vi "Temperature On Error.vi"() -> ()   [LabVIEW 2012, in "Phidget Temperature Sensor.lvlib"]
uses:
  <instrlib>/Phidgets/Phidget Temperature Sensor/Phidget Temperature Sensor.lvlib
  <instrlib>/Phidgets/Phidget Temperature Sensor/Public/TemperatureSensorStart.vi
  <instrlib>/Phidgets/Phidget Temperature Sensor/Public/TemperatureSensorClose.vi
  <instrlib>/Phidgets/Phidget Common/Phidget Common.lvlib
panel:
  out "Serial Number Return":i32
  in  "Device Info":T1={"Serial Number"=-1, "Channel"=0, "Port"=0}
  out "error out":errorcluster
  in  "stop":bool
  out "ErrorString":string
  out "ErrorCode":i32
  # "This will receive the error generated if a reading is out of range"
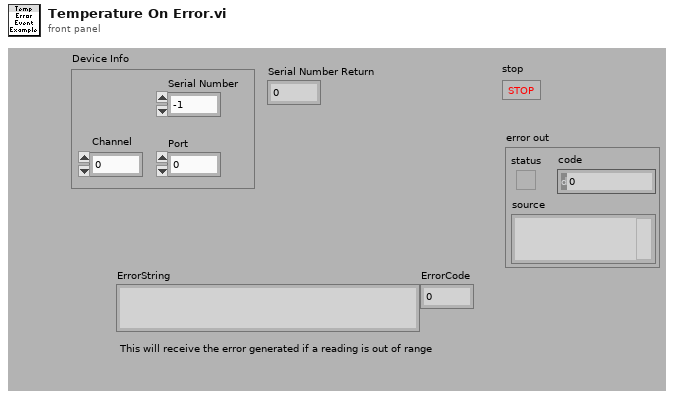
[diagram p1: front panel]
types:
  T1 = cluster{"Serial Number":i32, "Channel":i32, "Port":i32}
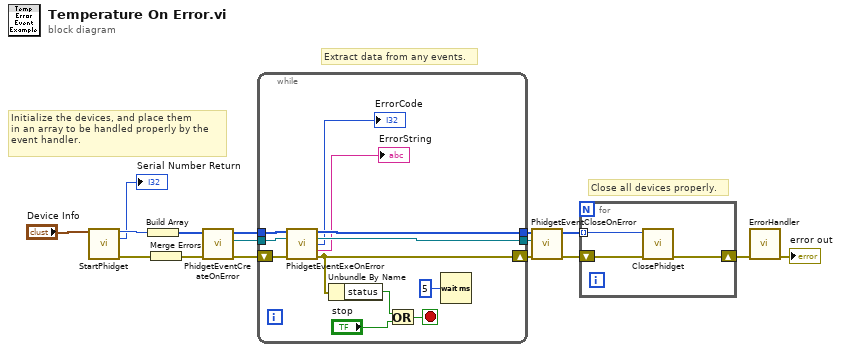
[diagram p0: block diagram]
diagram:
  # "Close all devices properly."
  # "Extract data from any events."
  # "Initialize the devices, and place them\nin an array to be handled properly by the\nevent handler."
  n1 = call-poly <instrlib>:"StartPhidget.vi"("Device Info"="Device Info") -> ("Phidget ID"=w5:u64, "Serial Number Return"=→"Serial Number Return":i32, "error out"=w1:errorcluster)  [unwired: 11 in, 1 out]
  n2 = Build Array(w5) -> (w16:u64[])
  n3 = Merge Errors(w1) -> (w7:errorcluster)
  n4 = call <instrlib>:"PhidgetEventCreateOnError.vi"("error in (no error)"=w7, "Devices In"=w16) -> ("error out"=w9:errorcluster, "Event Registration Refnum"=w14:refnum<event-registration>, "Devices Out"=w15:u64[])  [unwired: 7 in]
  n5 = while {
    tunnel: w15 -> [w28]
    tunnel: w14 -> [w24]
    tunnel: [w27] -> w11
    shift-right: [w17] -> w10
    shift-left: w9 -> [w26]
    tunnel: [w20] -> w3
    stop <- w23 stop-if-true
    n6 = call <instrlib>:"PhidgetEventExeOnError.vi"("Devices In"=w28, "Event Registration Refnum In"=w24, "error in (no error)"=w26) -> ("Devices Out"=w20:u64[], "Event Registration Refnum Out"=w27:refnum<event-registration>, "ErrorCode"=→"ErrorCode":i32, "ErrorString"=→"ErrorString":string, "error out"=w17:errorcluster)  [unwired: 5 in, 3 out]
    n7 = Unbundle By Name(w17) -> ("status"=w21:bool)
    n8 = Or(x=w21, y="stop") -> (x .or. y?=w23:bool)
    n9 = Wait (ms)(milliseconds to wait=u32 5) -> ()  [unwired: 1 out]
  }
  n10 = call <instrlib>:"PhidgetEventCloseOnError.vi"("error in (no error)"=w10, "Event Registration Refnum In"=w11, "Devices In"=w3) -> ("error out"=w6:errorcluster, "Devices Out"=w4:u64[])  [unwired: 7 in]
  n11 = for {
    tunnel: w4 -> [w29] mode=indexing
    shift-right: [w31] -> w13
    shift-left: w6 -> [w30]
    n12 = call-poly <instrlib>:"ClosePhidget.vi"("error in"=w30, "Device In"=w29) -> ("error out"=w31:errorcluster)  [unwired: 9 in]
  }
  n13 = call <instrlib>:"ErrorHandler.vi"("error in"=w13) -> ("error out"=→"error out":errorcluster)  [unwired: 9 in, 1 out]
